vi "LinkNodes.vi"(8 "error in (no error)":errorcluster, 9 "LinkInfo":T1, 10 "Child in":refnum<data-value>, 11 "Parent in":refnum<data-value>) -> (0 "error out":errorcluster, 1 "ignored":bool, 2 "Child out":refnum<data-value>, 3 "Parent out":refnum<data-value>)   [LabVIEW 2009, in "Tree.lvclass"]
doc: "Links a parent node and a child node. You can choose where to link it via the LinkInfo input."
uses:
  Tree.lvclass
  TreeNode/TreeNode.lvclass
  LinkInfo.ctl
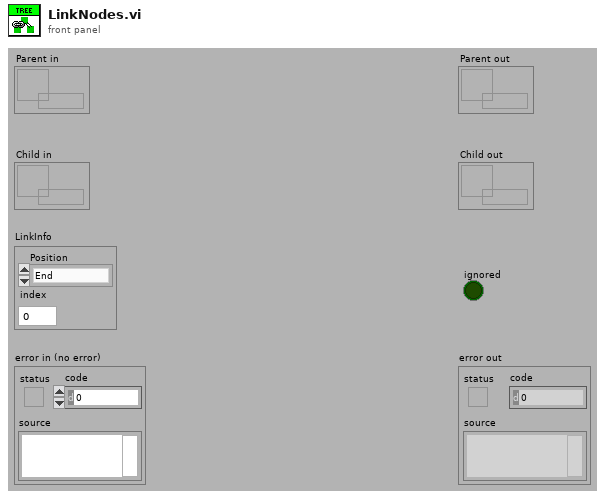
[diagram p1: front panel]
types:
  T1 = typedef "Tree.lvclass/LinkInfo.ctl" = cluster{"Position":enum16{"End", "Front", "Index"}, "index":i32}
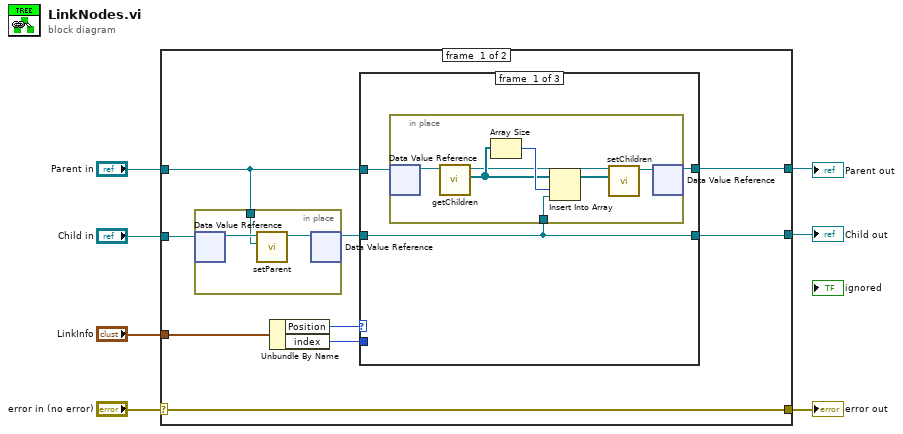
[diagram p0: block diagram]
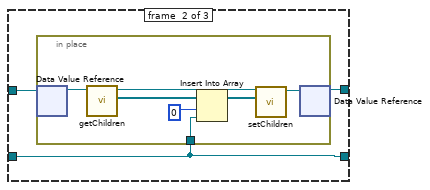
[diagram p2: hidden frame]
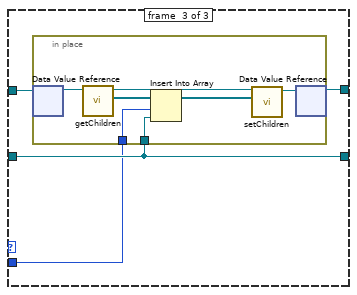
[diagram p3: hidden frame]
diagram:
  n1 = case shown="No Error" "error in (no error)" {
    selector: "error in (no error)" -> [w16 w53]
    tunnel: [w16 w53] -> w6
    tunnel: "LinkInfo" -> [w15 _]
    tunnel: "Parent in" -> [w10 w52]
    tunnel: "Child in" -> [w12 w51]
    tunnel: [w9 w52] -> w2
    tunnel: [w8 w51] -> w1
    frame #0 {
      n2 = in-place {
        in-place-border: w10 -> [w17]
        n3 = in-place-dvr #1(w12) -> (w19:refnum<class "TreeNode.lvclass">)  [unwired: 1 out]
        n4 = call "setParent.vi"("Parent"=w17, "TreeNode in"=w19) -> ("TreeNode out"=w18:refnum<class "TreeNode.lvclass">)  [unwired: 8 in, 1 out]
        n5 = in-place-dvr #1(w18) -> (w11:refnum<data-value>)  [unwired: 1 out]
      }
      n6 = Unbundle By Name(w15) -> ("Position"=w14:enum16{"End", "Front", "Index"}, "index"=w13:i32)
      n7 = case shown="\"Index\"" w14 {
        tunnel: w13 -> [_ _ w41]
        tunnel: w11 -> [w20 w30 w42]
        tunnel: w10 -> [w22 w32 w43]
        tunnel: [w21 w31 w40] -> w9
        tunnel: [w20 w30 w42] -> w8
        frame #0 {
          n8 = in-place {
            in-place-border: w20 -> [w27]
            n9 = in-place-dvr #2(w22) -> (w29:refnum<class "TreeNode.lvclass">)  [unwired: 1 out]
            n10 = call "getChildren.vi"("TreeNode in"=w29) -> ("Children"=w26:refnum<data-value>[], "TreeNode out"=w24:refnum<class "TreeNode.lvclass">)  [unwired: 8 in, 1 out]
            n11 = Array Size(array=w26) -> (size(s)=w28:i32)
            n12 = Insert Into Array(array=w26, index=w28, new element=w27) -> (w25:refnum<data-value>[])
            n13 = call "setChildren.vi"("Children"=w25, "TreeNode in"=w24) -> ("TreeNode out"=w23:refnum<class "TreeNode.lvclass">)  [unwired: 8 in, 1 out]
            n14 = in-place-dvr #2(w23) -> (w21:refnum<data-value>)  [unwired: 1 out]
          }
        }
        frame #1 {
          n15 = in-place {
            in-place-border: w30 -> [w38]
            n16 = in-place-dvr #3(w32) -> (w39:refnum<class "TreeNode.lvclass">)  [unwired: 1 out]
            n17 = call "getChildren.vi"("TreeNode in"=w39) -> ("Children"=w33:refnum<data-value>[], "TreeNode out"=w36:refnum<class "TreeNode.lvclass">)  [unwired: 8 in, 1 out]
            n18 = Insert Into Array(array=w33, index=0, new element=w38) -> (w37:refnum<data-value>[])
            n19 = call "setChildren.vi"("Children"=w37, "TreeNode in"=w36) -> ("TreeNode out"=w35:refnum<class "TreeNode.lvclass">)  [unwired: 8 in, 1 out]
            n20 = in-place-dvr #3(w35) -> (w31:refnum<data-value>)  [unwired: 1 out]
          }
        }
        frame #2 {
          n21 = in-place {
            in-place-border: w42 -> [w49]
            in-place-border: w41 -> [w45]
            n22 = in-place-dvr #4(w43) -> (w50:refnum<class "TreeNode.lvclass">)  [unwired: 1 out]
            n23 = call "getChildren.vi"("TreeNode in"=w50) -> ("Children"=w48:refnum<data-value>[], "TreeNode out"=w47:refnum<class "TreeNode.lvclass">)  [unwired: 8 in, 1 out]
            n24 = Insert Into Array(array=w48, index=w45, new element=w49) -> (w44:refnum<data-value>[])
            n25 = call "setChildren.vi"("Children"=w44, "TreeNode in"=w47) -> ("TreeNode out"=w46:refnum<class "TreeNode.lvclass">)  [unwired: 8 in, 1 out]
            n26 = in-place-dvr #4(w46) -> (w40:refnum<data-value>)  [unwired: 1 out]
          }
        }
      }
    }
    frame #1 {
    }
  }
  "error out" <- w6
  "Parent out" <- w2
  "Child out" <- w1
